vi "Script_Excit_Extract_Table_From_Text.vi"(8 "error in (no error)":errorcluster, 10 "Excit Text":string="script  excit1wfm\n    wait until scriptTrigger0\n    generate E1TwoSwift0p5f250p0to600p0a70and700p0to1000p0a50d1200fs10\n    generate E2Chirp3p5f250p0to1000p0a50d800fs10\n    generate E3TwoSwift0p5f250p0to600p0a70and700p0to1000p0a50d1200fs10\n    generate E4Chirp3p5f250p0to1000p0a50d800fs10\n    generate E5Chirp3p5f250p0to1000p0a50d800fs40\nend script", 11 "Number of Excitations":u16=3) -> (0 "error out":errorcluster, 2 "Table of Wfms":string[](array[string]), 3 "EXCIT Table":T1={"Number of Excits"=0, "Number of Ejects"=0, "Sampling Frequency"=0.0, "Waveforms Table"=[["Excit1", "name", "Swift", "0.5", "1200", "70", "150", "550", "0", "0", "0"]]})   [LabVIEW 2020]
uses:
  controls/EXCIT_Table.ctl
panel:
  in  "EXCIT Table":T1={"Number of Excits"=0, "Number of Ejects"=0, "Sampling Frequency"=0.0, "Waveforms Table"=[["Excit1", "name", "Swift", "0.5", "1200", "70", "150", "550", "0", "0", "0"]]}
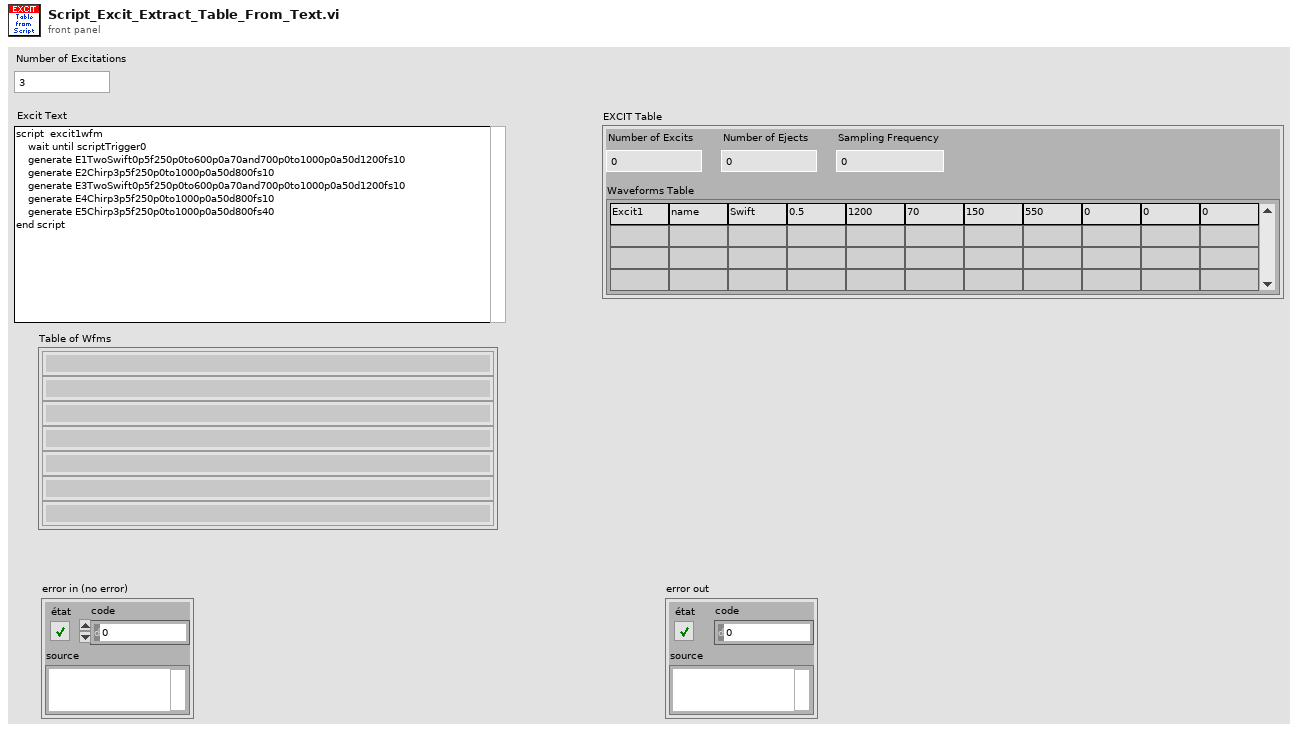
[diagram p1: front panel]
types:
  T1 = typedef "EXCIT_Table.ctl" = cluster{"Number of Excits":u16, "Number of Ejects":u16, "Sampling Frequency":dbl, "Waveforms Table":string[][]}
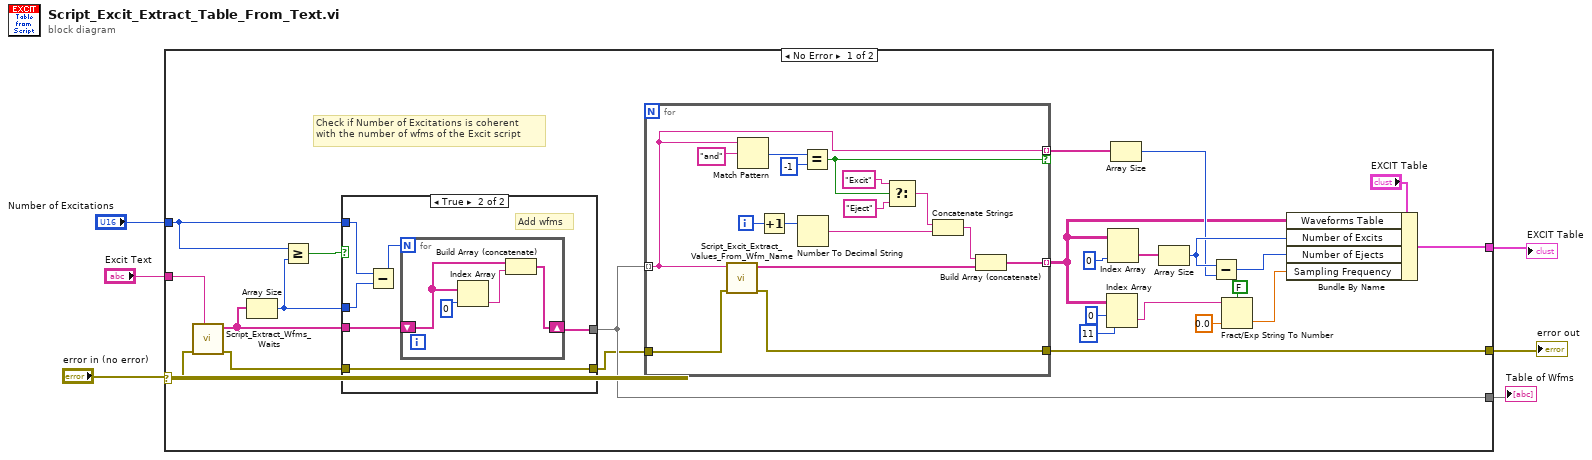
[diagram p0: block diagram]
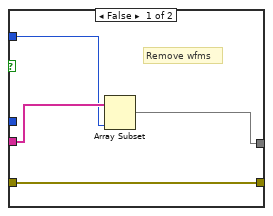
[diagram p2: hidden frame]
diagram:
  n1 = case shown="No Error" "error in (no error)" {
    selector: "error in (no error)" -> [w29 w62]
    tunnel: [w27 w62] -> w5
    tunnel: "Excit Text" -> [w30 _]
    tunnel: [w28 _] -> w3
    tunnel: [w13 _] -> w2
    tunnel: "Number of Excitations" -> [w10 _]
    frame No Error {
      # "Check if Number of Excitations is coherent\nwith the number of wfms of the Excit script"
      n2 = call "Script_Extract_Wfms_Waits.vi"("Script Text"=w30, "error in (no error)"=w29) -> ("error out"=w8:errorcluster, "Table of Loaded Wfms"=w12:string[])  [unwired: 6 in, 2 out]
      n3 = Array Size(array=w12) -> (size(s)=w9:i32)
      n4 = Greater Or Equal?(x=w10, y=w9) -> (x >= y?=w11:bool)
      n5 = case shown="True" w11 {
        tunnel: w12 -> [w35 w38]
        tunnel: [w33 w37] -> w13
        tunnel: w10 -> [w34 w40]
        tunnel: w9 -> [_ w39]
        tunnel: w8 -> [w32 w36]
        tunnel: [w32 w36] -> w7
        frame False {
          # "Remove wfms"
          n6 = Array Subset(array=w35, length=w34) -> (w33:string[])  [unwired: 1 in]
        }
        frame True {
          # "Add wfms"
          n7 = Subtract(x=w40, y=w39) -> (x-y=w41:i32)
          n8 = for {
            N: w41 -> [_]
            shift-right: [w42] -> w37
            shift-left: w38 -> [w45]
            n9 = Index Array(array=w45, index=0 ("indice")) -> (element=w43:string)
            n10 = Build Array (concatenate)(w45, w43) -> (w42:string[])
          }
        }
      }
      n11 = for {
        tunnel: w13 -> [w46] mode=indexing
        tunnel: [w56] -> w19 mode=indexing
        tunnel: w7 -> [w54]
        tunnel: [w53] -> w27
        tunnel: [w46] -> w22 mode=indexing if=w47
        i -> [w60]
        n12 = call "Script_Excit_Extract_Values_From_Wfm_Name.vi"("error in (no error)"=w54, "Excit Wfm String"=w46) -> ("error out"=w53:errorcluster, "Excit Wfm Values"=w57:string[])  [unwired: 8 in]
        n13 = Match Pattern(string=w46, regular expression="and" ("expression régulière")) -> (offset past match=w52:i32)  [unwired: 1 in, 3 out]
        n14 = Increment(x=w60) -> (x+1=w59:i32)
        n15 = Number To Decimal String(number=w59) -> (decimal integer string=w61:string)  [unwired: 1 in]
        n16 = Equal?(x=w52, y=-1) -> (x = y?=w47:bool)
        n17 = Select(t="Excit" ("chaîne"), s=w47, f="Eject" ("chaîne")) -> (s? t:f=w48:string)
        n18 = Concatenate Strings(w48, w61) -> (w58:string)
        n19 = Build Array (concatenate)(w58, w57) -> (w56:string[])
      }
      n20 = Index Array(array=w19, index (row)=0 ("indice (ligne)"), index (col)=11 ("indice désactivé (col)")) -> (element=w16:string)
      n21 = Index Array(array=w19, index (col)=0 ("indice désactivé (col)")) -> (element=w21:string[])  [unwired: 1 in]
      n22 = Array Size(array=w22) -> (size(s)=w24:i32)
      n23 = Array Size(array=w21) -> (size(s)=w25:i32)
      n24 = Subtract(x=w25, y=w24) -> (x-y=w23:i32)
      n25 = Fract/Exp String To Number(use system decimal point (T)=FALSE ("utiliser le séparateur décimal du système (V)"), string=w16, default (0 dbl)=0.0 ("valeur par défaut (0 DBL)")) -> (number=w20:dbl)  [unwired: 1 in, 1 out]
      n26 = Bundle By Name(cluster="EXCIT Table", "Waveforms Table"=w19, "Number of Excits"=w25, "Number of Ejects"=w23, "Sampling Frequency"=w20) -> (w28:T1)
    }
    frame Error {
    }
  }
  "error out" <- w5
  "EXCIT Table" <- w3
  "Table of Wfms" <- w2
